vi "Data Trim Module.vi"(7 "#pixels to save":i32=300, 8 "error in":errorcluster, 9 "start pixel":i32, 10 "#A-lines":i32=2048, 11 "1D Array in":u16[](array[numeric])) -> (0 "error out":errorcluster, 2 "array for saving":u16[](array[numeric]))   [LabVIEW 2018]
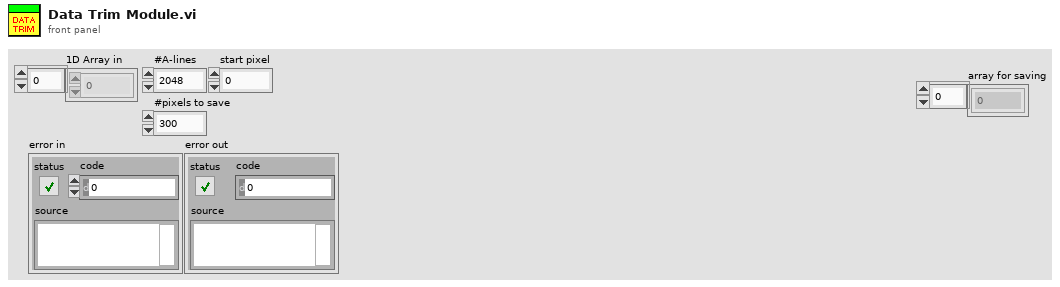
[diagram p1: front panel]
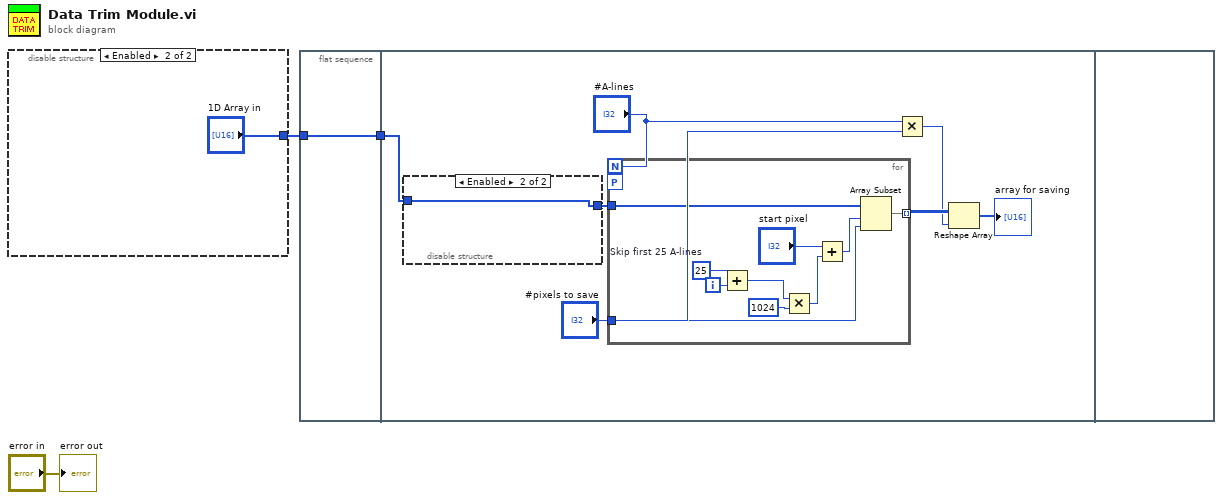
[diagram p0: block diagram]
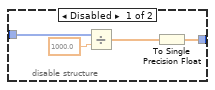
[diagram p2: hidden frame]
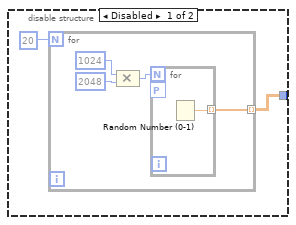
[diagram p3: hidden frame]
diagram:
  n1 = disable-structure shown="Enabled" {
    disable-tunnel: [w4 "1D Array in"] -> w1
    frame Disabled {
      n2 = for {
        N: 20 -> [_]
        tunnel: [w6] -> w4 mode=indexing
        n3 = Compound Arithmetic op=MULTIPLY(1024, 2048) -> (w7:i32)
        n4 = for {
          N: w7 -> [_]
          tunnel: [w10] -> w6 mode=indexing
          workers-P: _ -> [_]
          n5 = Random Number (0-1)() -> (number: 0 to 1=w10:dbl)
        }
      }
    }
    frame Enabled {
    }
  }
  n6 = flat-sequence {
    tunnel: w1 -> [w12]
    tunnel: [w12] -> w3
    tunnel: w3 -> [w19]
    frame #0 {
    }
    frame #1 {
      n7 = disable-structure shown="Enabled" {
        disable-tunnel: w19 -> [w33 w34]
        disable-tunnel: [w30 w34] -> w18
        frame Disabled {
          n8 = Divide(x=w33, y=sgl 1000.0) -> (x/y=w31:sgl[])
          n9 = To Single Precision Float(number=w31) -> (single precision float=w30:sgl[])
        }
        frame Enabled {
        }
      }
      n10 = for {
        N: "#A-lines" -> [_]
        tunnel: w18 -> [w28]
        workers-P: _ -> [_]
        tunnel: [w27] -> w17 mode=indexing
        tunnel: "#pixels to save" -> [w26]
        i -> [w21]
        w22 = 25  # Skip first 25 A-lines
        n11 = Add(x=w22, y=w21) -> (x+y=w20:i32)
        n12 = Multiply(x=w20, y=1024) -> (x*y=w24:i32)
        n13 = Add(x="start pixel", y=w24) -> (x+y=w23:i32)
        n14 = Array Subset(array=w28, index=w23, length=w26) -> (w27:u16[])
      }
      n15 = Multiply(x="#A-lines", y="#pixels to save") -> (x*y=w14:i32)
      n16 = Reshape Array(w17, w14) -> (→"array for saving":u16[])
    }
    frame #2 {
    }
  }
  "error out" <- "error in"
